vi "2022-InitGlobalConstants.vi"(8 "error in (no error)":errorcluster, 11 "localConstantSpreadSheet":string[][](array[string])) -> (0 "error out":errorcluster)   [LabVIEW 2020]
uses:
  2020LabView/2020-Robot Global Data.vi
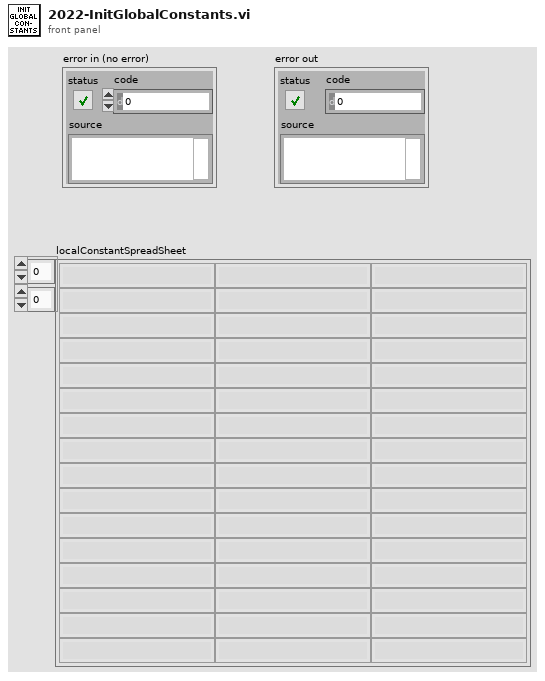
[diagram p1: front panel]
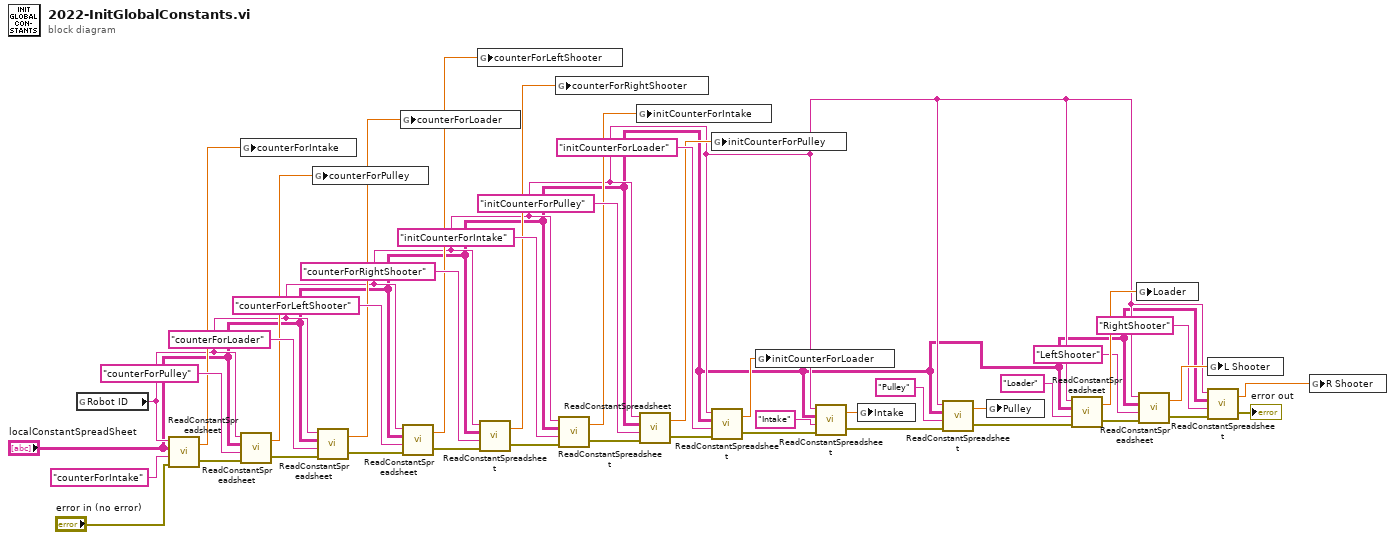
[diagram p0: block diagram]
diagram:
  n1 = global read "2020-Robot Global Data.vi" "Robot ID"() -> (w4:string)
  n2 = call "ReadConstantSpreadsheet.vi"("error in"="error in (no error)", "Constant"="counterForIntake" ("Motor ID"), "2020ConstantSpreadSheet"="localConstantSpreadSheet", "Robot ID"=w4) -> ("error out"=w14:errorcluster, "Constant Value"=w24:dbl)
  n3 = global write "2020-Robot Global Data.vi" "counterForIntake"(w24) -> ()
  n4 = call "ReadConstantSpreadsheet.vi"("error in"=w14, "Constant"="counterForPulley" ("Motor ID"), "2020ConstantSpreadSheet"="localConstantSpreadSheet", "Robot ID"=w4) -> ("error out"=w16:errorcluster, "Constant Value"=w30:dbl)
  n5 = global write "2020-Robot Global Data.vi" "counterForPulley"(w30) -> ()
  n6 = call "ReadConstantSpreadsheet.vi"("error in"=w16, "Constant"="counterForLoader" ("Motor ID"), "2020ConstantSpreadSheet"="localConstantSpreadSheet", "Robot ID"=w4) -> ("error out"=w12:errorcluster, "Constant Value"=w23:dbl)
  n7 = global write "2020-Robot Global Data.vi" "counterForLoader"(w23) -> ()
  n8 = call "ReadConstantSpreadsheet.vi"("error in"=w12, "Constant"="counterForLeftShooter" ("Motor ID"), "2020ConstantSpreadSheet"="localConstantSpreadSheet", "Robot ID"=w4) -> ("error out"=w13:errorcluster, "Constant Value"=w31:dbl)
  n9 = global write "2020-Robot Global Data.vi" "counterForLeftShooter"(w31) -> ()
  n10 = call "ReadConstantSpreadsheet.vi"("error in"=w13, "Constant"="counterForRightShooter" ("Motor ID"), "2020ConstantSpreadSheet"="localConstantSpreadSheet", "Robot ID"=w4) -> ("error out"=w21:errorcluster, "Constant Value"=w25:dbl)
  n11 = global write "2020-Robot Global Data.vi" "counterForRightShooter"(w25) -> ()
  n12 = call "ReadConstantSpreadsheet.vi"("error in"=w21, "Constant"="initCounterForIntake" ("Motor ID"), "2020ConstantSpreadSheet"="localConstantSpreadSheet", "Robot ID"=w4) -> ("error out"=w11:errorcluster, "Constant Value"=w32:dbl)
  n13 = global write "2020-Robot Global Data.vi" "initCounterForIntake"(w32) -> ()
  n14 = call "ReadConstantSpreadsheet.vi"("error in"=w11, "Constant"="initCounterForPulley" ("Motor ID"), "2020ConstantSpreadSheet"="localConstantSpreadSheet", "Robot ID"=w4) -> ("error out"=w20:errorcluster, "Constant Value"=w26:dbl)
  n15 = global write "2020-Robot Global Data.vi" "initCounterForPulley"(w26) -> ()
  n16 = call "ReadConstantSpreadsheet.vi"("error in"=w20, "Constant"="initCounterForLoader" ("Motor ID"), "2020ConstantSpreadSheet"="localConstantSpreadSheet", "Robot ID"=w4) -> ("error out"=w15:errorcluster, "Constant Value"=w29:dbl)
  n17 = global write "2020-Robot Global Data.vi" "initCounterForLoader"(w29) -> ()
  n18 = call "ReadConstantSpreadsheet.vi"("error in"=w15, "Constant"="Intake" ("Motor ID"), "2020ConstantSpreadSheet"="localConstantSpreadSheet", "Robot ID"=w4) -> ("error out"=w10:errorcluster, "Constant Value"=w27:dbl)
  n19 = global write "2020-Robot Global Data.vi" "Intake"(w27) -> ()
  n20 = call "ReadConstantSpreadsheet.vi"("error in"=w10, "Constant"="Pulley" ("Motor ID"), "2020ConstantSpreadSheet"="localConstantSpreadSheet", "Robot ID"=w4) -> ("error out"=w19:errorcluster, "Constant Value"=w42:dbl)
  n21 = global write "2020-Robot Global Data.vi" "Pulley"(w42) -> ()
  n22 = call "ReadConstantSpreadsheet.vi"("error in"=w19, "Constant"="Loader" ("Motor ID"), "2020ConstantSpreadSheet"="localConstantSpreadSheet", "Robot ID"=w4) -> ("error out"=w9:errorcluster, "Constant Value"=w17:dbl)
  n23 = global write "2020-Robot Global Data.vi" "Loader"(w17) -> ()
  n24 = call "ReadConstantSpreadsheet.vi"("error in"=w9, "Constant"="LeftShooter" ("Motor ID"), "2020ConstantSpreadSheet"="localConstantSpreadSheet", "Robot ID"=w4) -> ("error out"=w5:errorcluster, "Constant Value"=w7:dbl)
  n25 = global write "2020-Robot Global Data.vi" "L Shooter"(w7) -> ()
  n26 = call "ReadConstantSpreadsheet.vi"("error in"=w5, "Constant"="RightShooter" ("Motor ID"), "2020ConstantSpreadSheet"="localConstantSpreadSheet", "Robot ID"=w4) -> ("error out"=→"error out":errorcluster, "Constant Value"=w6:dbl)
  n27 = global write "2020-Robot Global Data.vi" "R Shooter"(w6) -> ()
